vi "Control.vi"() -> ()   [LabVIEW 2018]
uses:
  <vilib>/FPGAPlugInAG/cRIO-9039 (Sync)/niLvFpga_Open_cRIO-9039 (Sync).vi
  <vilib>/rvi/interface/common/dynamic/niFpgaDynamicAddResources.vi
  <vilib>/Utility/error.llb/Error Cluster From Error Code.vi
  <vilib>/rvi/errors/niLvFpgaAdjustHostInterfaceError.vi
  <vilib>/FPGAPlugInAG/Dynamic/niLvFpga_Close_Dynamic.vi
  <vilib>/rvi/interface/nirviOpenFPGA/nirviOpenFPGA.xnode
  NIFPGA/compilation/M1M3SupportFPGA.lvbitx
  M1M3SupportFPGA.vi
  <vilib>/rvi/interface/nirviReadWriteControl/nirviReadWriteControl.xnode
  <vilib>/rvi/interface/nirviMethod/nirviMethod.xnode
  <vilib>/rvi/interface/nirviCloseFPGA/nirviCloseFPGA.xnode
  <vilib>/rvi/interface/Simulation/niFpgaSimulationCallBeginRW.vi
  NiFpgaLv.dll
  <vilib>/FPGAPlugInAG/Dynamic/niLvFpga_WriteFifo_Dynamic.vi
  <vilib>/rvi/errors/niLvFpgaMergeErrorWithErrorCode.vi
panel:
  in  "Tab Control":enum32{"Commands", "Modbus"}(tab)
  in  "?":bool
  out "Failed":u64
  out "Commands":u64
  in  "Address":dbl
  in  "Port":i32(listbox)
  out "D Tx":u64
  out "D Rx":u64
  out "C Tx":u64
  out "C Rx":u64
  out "B Tx":u64
  out "B Rx":u64
  out "A Tx":u64
  out "A Rx":u64
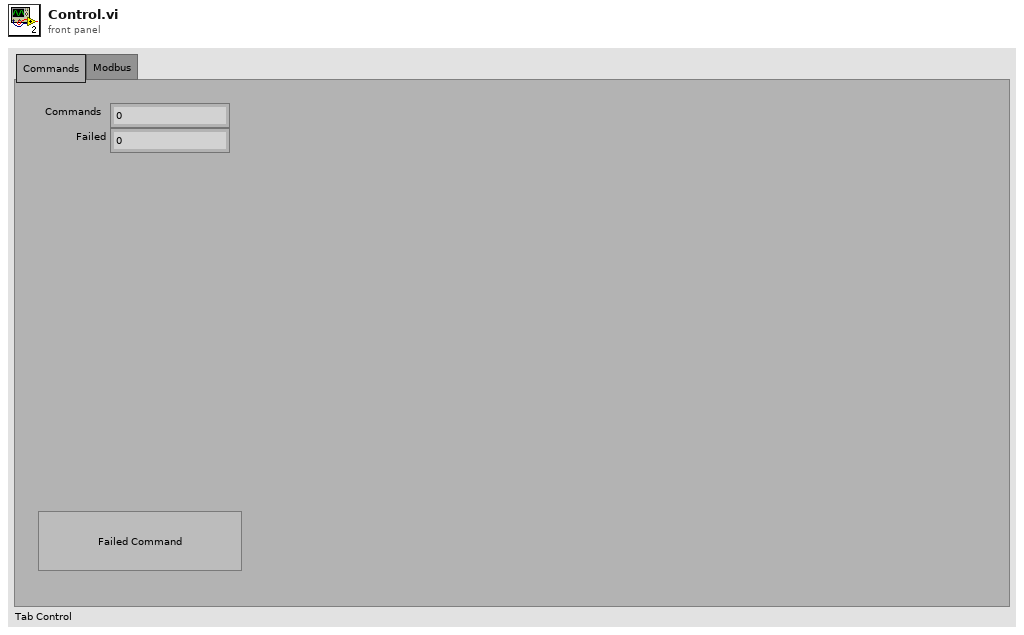
[diagram p1: front panel]
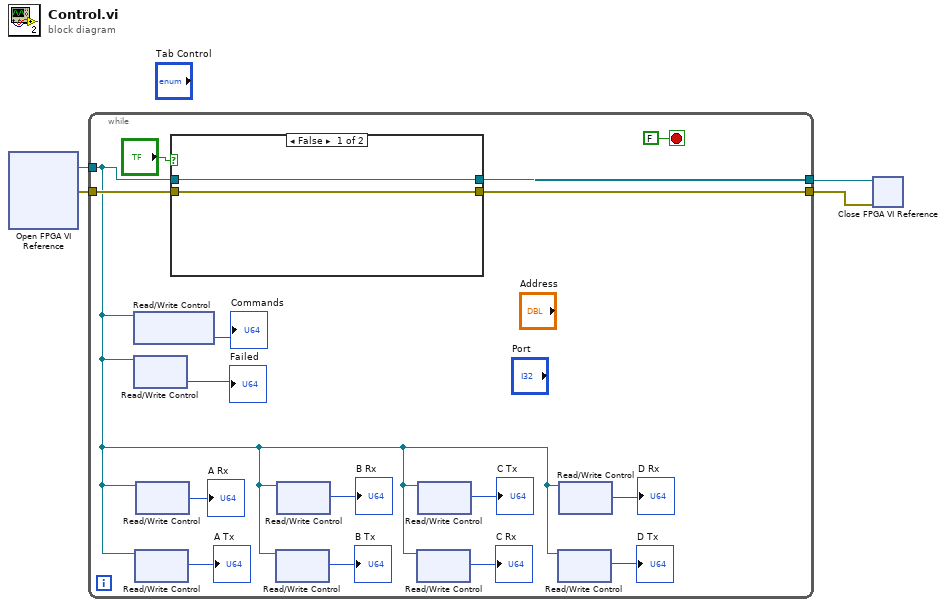
[diagram p0: block diagram]
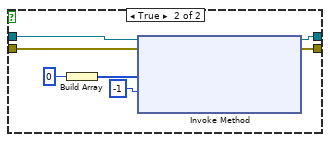
[diagram p2: hidden frame]
diagram:
  n1 = xnode "Open FPGA VI Reference"() -> ("FPGA VI Reference Out"=w4:refnum<k20>, "error out"=w3:errorcluster)  [unwired: 2 in]
  n2 = while {
    tunnel: w4 -> [w9]
    tunnel: w3 -> [w18]
    tunnel: [w17] -> w2
    tunnel: [w16] -> w1
    stop <- FALSE stop-if-true
    n3 = xnode "Read/Write Control"("FPGA VI Reference In"=w9) -> ("Commands"=→"Commands":u64)  [unwired: 1 in, 2 out]
    n4 = xnode "Read/Write Control"("FPGA VI Reference In"=w9) -> ("Failed"=→"Failed":u64)  [unwired: 1 in, 2 out]
    n5 = xnode "Read/Write Control"("FPGA VI Reference In"=w9) -> ("A Tx"=→"A Tx":u64)  [unwired: 1 in, 2 out]
    n6 = xnode "Read/Write Control"("FPGA VI Reference In"=w9) -> ("A Rx"=→"A Rx":u64)  [unwired: 1 in, 2 out]
    n7 = case shown="False" "?" {
      tunnel: w9 -> [w22 w28]
      tunnel: w18 -> [w21 w25]
      tunnel: [w22 w24] -> w17
      tunnel: [w21 w23] -> w16
      frame False {
      }
      frame True {
        n8 = Build Array(0) -> (w26:i32[])
        n9 = xnode "Invoke Method"("FPGA VI Reference In"=w28, "error in"=w25, "Data"=w26, "Timeout (ms)"=-1) -> ("FPGA VI Reference Out"=w24:refnum<k20>, "error out"=w23:errorcluster)  [unwired: 1 out]
      }
    }
    n10 = xnode "Read/Write Control"("FPGA VI Reference In"=w9) -> ("B Tx"=→"B Tx":u64)  [unwired: 1 in, 2 out]
    n11 = xnode "Read/Write Control"("FPGA VI Reference In"=w9) -> ("B Rx"=→"B Rx":u64)  [unwired: 1 in, 2 out]
    n12 = xnode "Read/Write Control"("FPGA VI Reference In"=w9) -> ("C Tx"=→"C Rx":u64)  [unwired: 1 in, 2 out]
    n13 = xnode "Read/Write Control"("FPGA VI Reference In"=w9) -> ("C Rx"=→"C Tx":u64)  [unwired: 1 in, 2 out]
    n14 = xnode "Read/Write Control"("FPGA VI Reference In"=w9) -> ("D Tx"=→"D Tx":u64)  [unwired: 1 in, 2 out]
    n15 = xnode "Read/Write Control"("FPGA VI Reference In"=w9) -> ("D Rx"=→"D Rx":u64)  [unwired: 1 in, 2 out]
  }
  n16 = xnode "Close FPGA VI Reference"("FPGA VI Reference In"=w2, "error in"=w1) -> ()  [unwired: 1 out]
